vi "Module_UI_TopLevel.vi"(8 "error in (no error)":errorcluster, 10 "Wait on Module(s) (\"\": none)":string, 11 "ConfigFiles Folder Path":path) -> (0 "error out":errorcluster)   [LabVIEW 2019, in "Module_UI_TopLevel.lvclass"]
doc: "JSMA Module Template - Top Level UI 0.2.0.4\nRob Humfeld - Jet Engineering\nCopyright (c) 2019, Jet Engineering"
uses:
  Module_UI_TopLevel.lvclass
  Private/Module_UI_TopLevel_JETLogo STYP.ctl
  XControl_Menu Button/Menu Button.xctl
  Private/Module_UI_TopLevel_SPRight STYP.ctl
  Private/Module_UI_TopLevel_SPBottom STYP.ctl
  Private/Module_UI_TopLevel_SPCenter STYP.ctl
  C:/Program Files/National Instruments/LabVIEW 2019/user.lib/Jet Engineering/JSMA/Libraries/jModule Class/jModule.lvclass
  Private/Module_UI_TopLevel_jMsgTx STYP.ctl
  <userlib>/Jet Engineering/JSMA/Libraries/jMsg_CORE/jMsg_JSMA_ApplicationShutdown/jMsg_JSMA_ApplicationShutdown.lvclass
  C:/Program Files/National Instruments/LabVIEW 2019/user.lib/Jet Engineering/JSMA/Libraries/jMsg Class/jMsg.lvclass
  <userlib>/JET Engineering/JSMA Standard Messages/jMsg_Sys_UIPanelOpen/jMsg_Sys_UIPanel_Open.lvclass
  <userlib>/Jet Engineering/JSMA GUISubPanel CORE/jMsgs/jMsg_Sys_GUIPanelDock/jMsg_GUISubPanel_Dock.lvclass
  <userlib>/Jet Engineering/JSMA GUISubPanel CORE/jMsgs/jMsg_Sys_GUIPanelUndocked/jMsg_GUISubPanel_Undocked.lvclass
  Private/Module_UI_TopLevel_jMsgRx STYP.ctl
  <userlib>/Jet Engineering/JSMA Standard Messages/jMsg_Sys_VersionInfo/jMsg_Sys_VersionInfo.lvclass
  Private/Module_UI_TopLevel_Status STYP.ctl
  Module_UI_TopLevel.lvclass/Module_UI_TopLevel.ctl
  <userlib>/Jet Engineering/JSMA/Libraries/jModule Class/jModule.lvclass/jModule.ctl
  <userlib>/Jet Engineering/JSMA/Libraries/jMsg Class/jMsg.lvclass/jMsg.ctl
  <userlib>/JET Engineering/JSMA Standard Messages/jMsg_Sys_UIPanelOpen/jMsg_Sys_UIPanel_Open.lvclass/jMsg_Sys_UIPanel_Open.ctl
  <userlib>/Jet Engineering/JSMA/Libraries/jMsg_CORE/jMsg_JSMA_Exception/jMsg_JSMA_Exception.lvclass/jMsg_JSMA_Exception.ctl
  <userlib>/Jet Engineering/JSMA/Libraries/jMsg_CORE/jMsg_JSMA_SubscriptionChange/jMsg_JSMA_SubscriptionChange.lvclass/jMsg_JSMA_SubscriptionChange.ctl
  <userlib>/Jet Engineering/JSMA/Libraries/jMsg_CORE/jMsg_Addressed/jMsg_Addressed.lvclass/jMsg_Addressed.ctl
  <userlib>/Jet Engineering/JSMA/Libraries/jMsg_CORE/jMsg_JSMA_ApplicationShutdown/jMsg_JSMA_ApplicationShutdown.lvclass/jMsg_JSMA_ApplicationShutdown.ctl
  <userlib>/Jet Engineering/JSMA GUISubPanel CORE/jMsgs/jMsg_Sys_GUIPanelDock/jMsg_GUISubPanel_Dock.lvclass/jMsg_GUISubPanel_Dock.ctl
  <userlib>/Jet Engineering/JSMA Standard Messages/jMsg_Sys_VersionInfo/jMsg_Sys_VersionInfo.lvclass/jMsg_Sys_VersionInfo.ctl
  <userlib>/Jet Engineering/JET_QSM/Code/Private/JET_QSM - Add State [String API].vi
  <userlib>/Jet Engineering/JET_QSM/Code/Private/JET_QSM - Add State to Front [String API].vi
  <userlib>/Jet Engineering/JSMA/Libraries/jModule Class/jModule - Set Static Timer.vi
  <userlib>/Jet Engineering/JSMA/Libraries/jModule Class/jModule - Set Periodic Timer.vi
  <userlib>/Jet Engineering/JSMA/Libraries/jMsg Class/(create) jMsg.vi
  <userlib>/Jet Engineering/JSMA/Libraries/jMsg_CORE/jMsg_JSMA_Exception/(create) jMsg_JSMA_Exception.vi
  <userlib>/Jet Engineering/JSMA/Libraries/jModule Class/jModule - Stats_Exception Count Increment.vi
  <userlib>/Jet Engineering/JSMA/Libraries/jModule Class/jModule - SimpleTx.vi
  <userlib>/Jet Engineering/JSMA/Libraries/jModule Class/jModule - Exception Enqueue.vi
  <userlib>/Jet Engineering/JSMA/Libraries/jMsg Class/Read No Listener Action.vi
  <userlib>/Jet Engineering/JSMA/Libraries/jModule Class/jModule - ExceptionBatchTx.vi
  <userlib>/Jet Engineering/JSMA/Libraries/jModule Class/jModule - Send to List.vi
  <userlib>/Jet Engineering/JSMA/Libraries/jModule Class/jModule - AddressedTx.vi
  <userlib>/Jet Engineering/JSMA/Libraries/jModule Class/jModule - Stats_Tx Count Increment.vi
  <userlib>/Jet Engineering/JSMA/Libraries/jMsg Class/Read Type.vi
  <userlib>/Jet Engineering/JSMA/Libraries/jMsg Class/Write SendID.vi
  <userlib>/Jet Engineering/JSMA/Libraries/jMsg Class/Read Name.vi
  <userlib>/Jet Engineering/JSMA/Libraries/jMasterTable_Subscription/jMasterTable_Subscription - Get Queue Type.vi
  <userlib>/Jet Engineering/JSMA/Libraries/jMsg Class/jMsg - Set Source.vi
  <userlib>/Jet Engineering/JSMA/Libraries/jMasterShutdownFlag/jFlag_MasterShutdown - Set.vi
  <userlib>/Jet Engineering/JSMA/Libraries/jModule Class/Read jMsgRx.vi
  <userlib>/Jet Engineering/JSMA/Libraries/Shared/JSMA_GetClassName.vi
  <userlib>/Jet Engineering/JSMA/Libraries/jMsg Class/Read Sent Time.vi
  <userlib>/Jet Engineering/JSMA/Libraries/jMsg Class/Read Source.vi
  <userlib>/Jet Engineering/JSMA/Libraries/jMasterTable_Subscription/jMasterTable_Subscription - Remove Module.vi
  <userlib>/Jet Engineering/JSMA/Libraries/jMsg Class/Write Source.vi
  <userlib>/Jet Engineering/JSMA/Libraries/jMsg_CORE/jMsg_JSMA_SubscriptionChange/(create) jMsg_JSMA_SubscriptionChange.vi
  <userlib>/Jet Engineering/JSMA/Libraries/jMasterTable_Subscription/jMasterTable_Subscription - Get Sub List.vi
  <userlib>/Jet Engineering/JSMA/Libraries/jMsg_CORE/jMsg_Addressed/Read Qualified Name.vi
  <userlib>/Jet Engineering/JSMA/Libraries/jMsg_CORE/jMsg_Addressed/Read RecvID.vi
  <userlib>/Jet Engineering/JSMA/Libraries/jMasterTable_Subscription/jMasterTable_Subscription - Get-Create Queue.vi
  <userlib>/Jet Engineering/JSMA/Libraries/jMasterTable_Message/jMasterTable_Message - Add jMsg.vi
  <userlib>/Jet Engineering/JSMA/Libraries/jMasterTable_Message/jMasterTable_Message - Get-Create Queue.vi
  <userlib>/Jet Engineering/JSMA/Libraries/jMsg_CORE/jMsg_JSMA_Exception/jMsg_JSMA_Exception.lvclass
  <userlib>/Jet Engineering/JSMA/Libraries/jMsg_CORE/jMsg_JSMA_SubscriptionChange/jMsg_JSMA_SubscriptionChange.lvclass
  <userlib>/Jet Engineering/JSMA/Libraries/jMsg_CORE/jMsg_Addressed/jMsg_Addressed.lvclass
  <vilib>/Utility/error.llb/Trim Whitespace.vi
  <vilib>/Utility/LVClass/Get LV Class Path.vi
  <userlib>/Jet Engineering/JSMA/Libraries/jMasterShutdownFlag/jFlag_MasterShutdown_FGV.vi
  <vilib>/Utility/error.llb/Error Cluster From Error Code.vi
  <userlib>/Jet Engineering/JSMA/Libraries/jModule Class/Read RxQueue.vi
  <userlib>/Jet Engineering/JSMA/Libraries/jSubscription Class/jSubscription.lvclass
  <userlib>/Jet Labs/JET Panel/JETPanel.lvclass
  <userlib>/Jet Engineering/JSMA/Libraries/jModule Class/jModule.lvclass
  <userlib>/Jet Engineering/JSMA/Libraries/jMasterShutdownFlag/jFlag_MasterShutdown.lvclass
  <userlib>/Jet Engineering/JSMA/Libraries/jMsg Class/jMsg.lvclass
panel:
  out "Center":T1=enum."Module_SP_CenterBlank#5"
  out "Bottom":T2=enum."Module_SP_BottomBlank#6"
  out "Right":T3=enum."Module_SP_RightBlank#7"
  out "Menu Level":string
  out "Menu Button":string
  out "String":string
  out "TCPStats":string
  out "FPGA":string caption="FPGA IO:"
  out "Host":string caption="Host PC:"
  in  "Menu":T4(xcontrol)
  in  "JET":T5
  out "currentDateTime":dbl format="%<%m/%d/%y %H:%M:%S>T"
  in  "exit?":bool
  out "winSizer 2":string="W"
  out "winSizer 1":string="W"
  out "Recent states before Error (with tick counts) 2":string="0.167 sec ago: VI Initialize\n0.167 sec ago: Window Open\n0.110 sec ago: Control Update\n0.110 sec ago: Indicator Update\n0.000 sec ago: Error Handler\r\n"
  out "Header":bool
  out "JETLogo":bool
  # "LOGO"
  # "LOGO"
  # "Project Name"
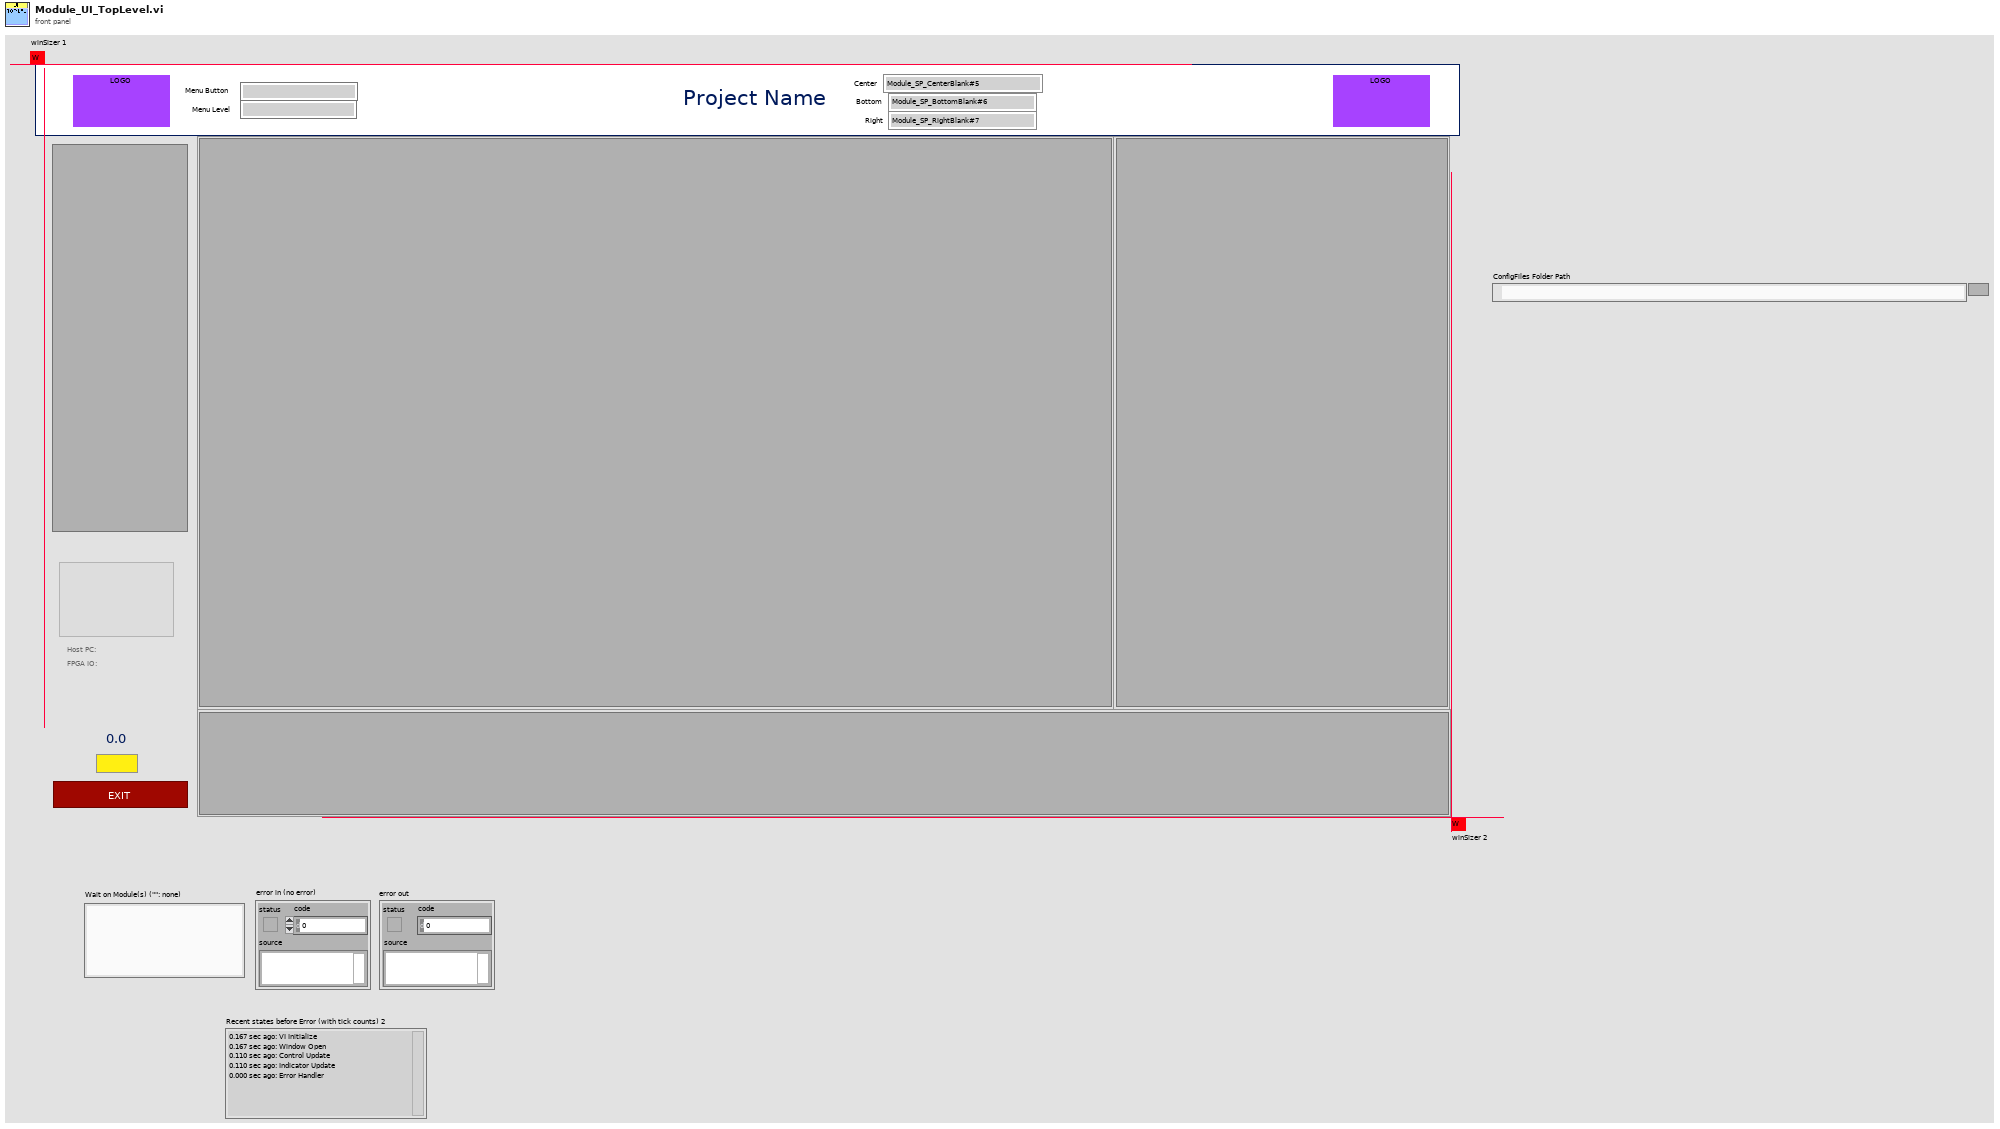
[diagram p1: front panel]
types:
  T1 = typedef "Module_UI_TopLevel.lvclass/Module_UI_TopLevel_SPCenter STYP.ctl" = enum16{"Module_SP_GameDisplay#0", "Module_SP_CenterBlank#5", "Module_SP_SALSignalConfig#4", "Module_SP_TestConfiguration#10", "Module_SP_TestExecution#9"}
  T2 = typedef "Module_UI_TopLevel.lvclass/Module_UI_TopLevel_SPBottom STYP.ctl" = enum16{"Module_SP_GameStats#2", "Module_SP_BottomBlank#6", "Module_SP_StatusRibbon#8"}
  T3 = typedef "Module_UI_TopLevel.lvclass/Module_UI_TopLevel_SPRight STYP.ctl" = enum16{"Module_SP_GameLeaderboard#1", "Module_SP_RightBlank#7", "Module_SP_SystemEventLog"}
  T4 = cluster{"Button Pressed":string, "Level":string, "Menu Config":variant}
  T5 = typedef "Module_UI_TopLevel.lvclass/Module_UI_TopLevel_JETLogo STYP.ctl" = bool
  T6 = typedef "Module_UI_TopLevel.lvclass/Module_UI_TopLevel_jMsgRx STYP.ctl" = cluster{"Msg_Sys_VersionInfo":refnum<class "jMsg_Sys_VersionInfo.lvclass">, "jMsg_GUISubPanel_Dock":refnum<class "jMsg_GUISubPanel_Dock.lvclass">}
  T7 = typedef "Module_UI_TopLevel.lvclass/Module_UI_TopLevel_jMsgTx STYP.ctl" = cluster{"jMsg_JSMA_ApplicationShutdown":refnum<class "jMsg_JSMA_ApplicationShutdown.lvclass">, "jMsg_Sys_UIPanel_Open":refnum<class "jMsg_Sys_UIPanel_Open.lvclass">, "jMsg_GUISubPanel_Dock":refnum<class "jMsg_GUISubPanel_Dock.lvclass">, "jMsg_GUISubPanel_Undocked":refnum<class "jMsg_GUISubPanel_Undocked.lvclass">}
  T8 = typedef "Module_UI_TopLevel.lvclass/Module_UI_TopLevel_Status STYP.ctl" = cluster{"VI":cluster{"error":errorcluster, "isExiting?":bool}, "UI":cluster{"SP_center":cluster{"refnum":refnum<vi>, "ActivePanel":T1}, "SP_bottom":cluster{"refnum":refnum<vi>, "ActivePanel":T2}, "SP_right":cluster{"refnum":refnum<vi>, "ActivePanel":T3}}, "TCPConnected?":bool}
  T9 = typedef "JET_QSM_Refnum STYP.ctl" = cluster{"state":cluster{"queue":refnum<queue>, "idle":string, "error":string, "STOP":string}, "debug":cluster{"enabled?":bool, "queue":refnum<queue>}, "Invalid.option":T10, "QSM.Name":string}
  T10 = typedef "JET_QSM_InvalidOption STYP.ctl" = enum16{"Ignore", "Dialog", "Error"}
  T11 = typedef "eventvkey.ctl" = enum16{"ASCII", "Enter", "Return", "Shift", "Ctrl", "Alt", "Cmd", "Opt", "Caps", "NumLock", "Clear", "Break", "Up", "Down", "Left", "Right", "Insert", "Delete", "Home", "End", "PageUp", "PageDown", "Escape", "Help", "Pause", "ScrollLock", "F1", "F2", "F3", "F4", "F5", "F6", "F7", "F8", "F9", "F10", "F11", "F12", "F13", "F14", "F15", "F16", "F17", "F18", "F19", "F20", "F21", "F22", "F23", "F24", "Play", "VolumeUp", "VolumeDown", "Mute", "Two Byte Char"}
  T12 = cluster{"Shift":bool, "Ctrl":bool, "Alt":bool, "Cmd":bool, "Opt":bool}
  T13 = typedef "JET_QSM_Element STYP.ctl" = cluster{"state":string, "data":variant, "comment":string}
  T14 = typedef "JSMAjMsg_Standard.lvlib/jMsg_Sys_VersionInfo.lvclass/VersionInfo STYP.ctl" = cluster{"ID":string, "Version":string, "Date":string}
  T15 = typedef "jSWCfg_SoftwareInfo STYP.ctl" = cluster{"target ID":string, "version":string, "releaseDate":string}
  T16 = enum8{"Enabled", "Disabled", "Disabled and Grayed Out"}
  T17 = typedef "jSWCfg_PROPERTIES STYP.ctl" = cluster{"SoftwareID":string, "SoftwareInfo.array":T15[]}
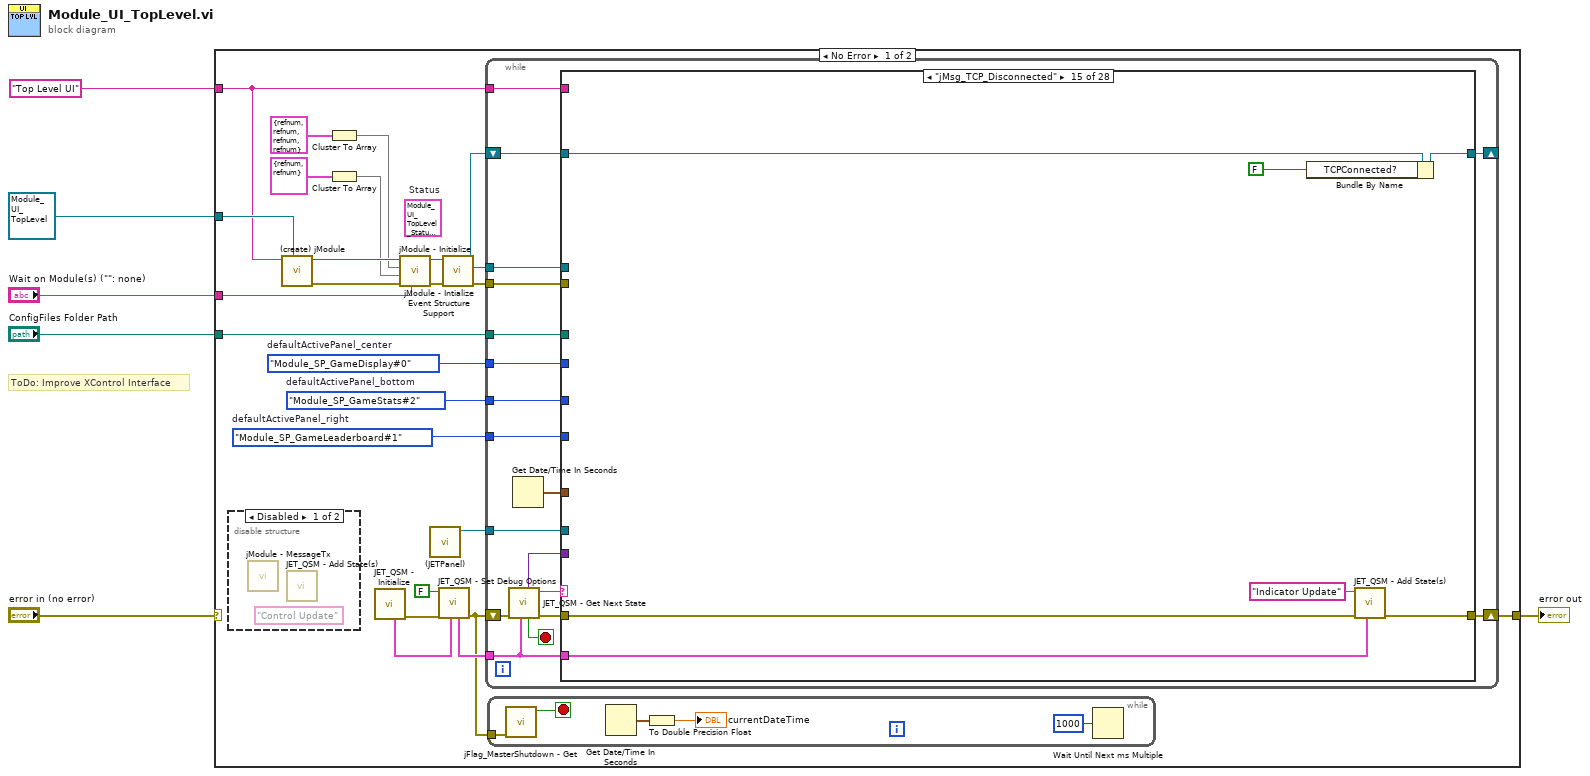
[diagram p0: block diagram]
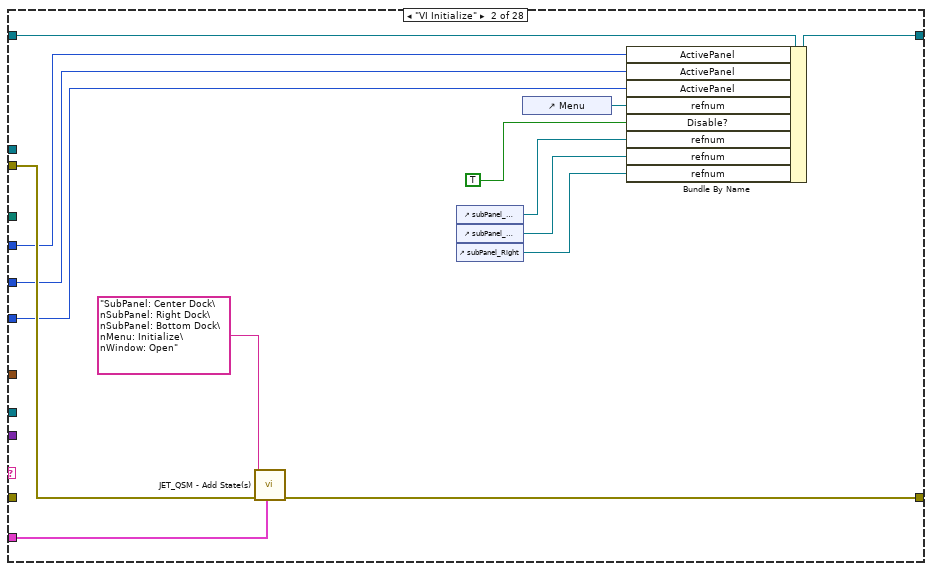
[diagram p4: hidden frame]
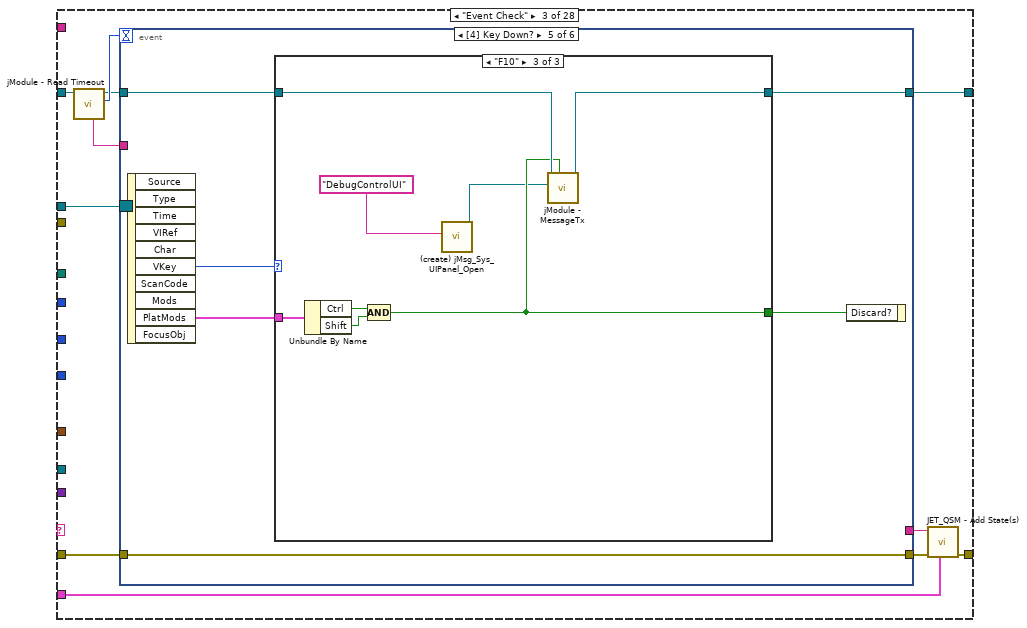
[diagram p5: hidden frame]
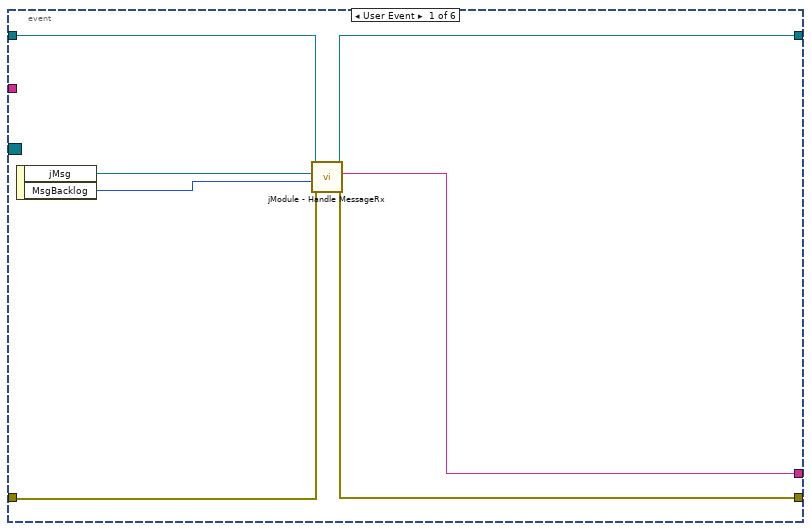
[diagram p6: hidden frame]
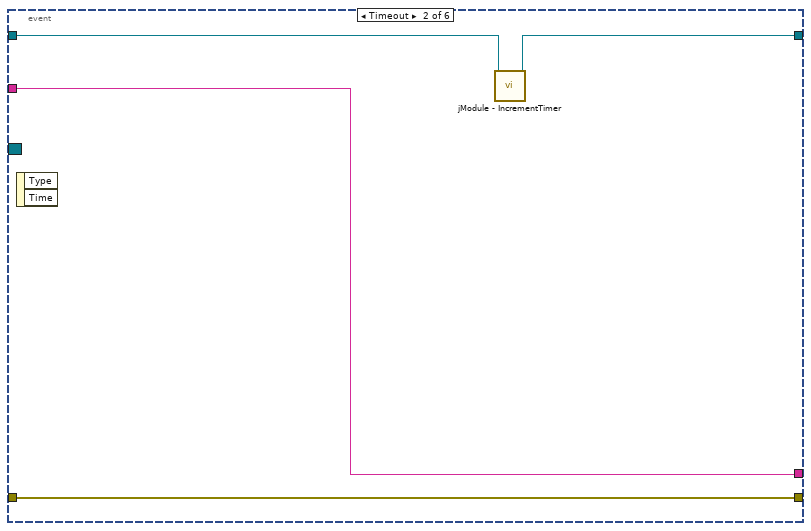
[diagram p7: hidden frame]
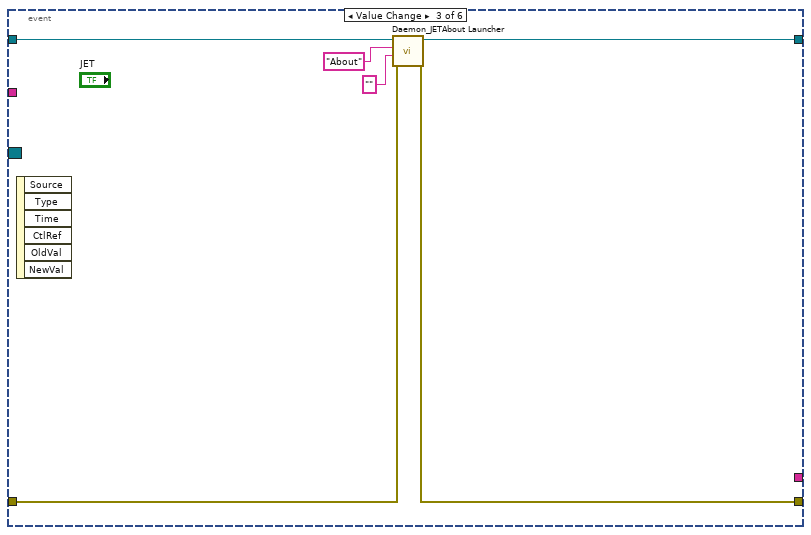
[diagram p8: hidden frame]
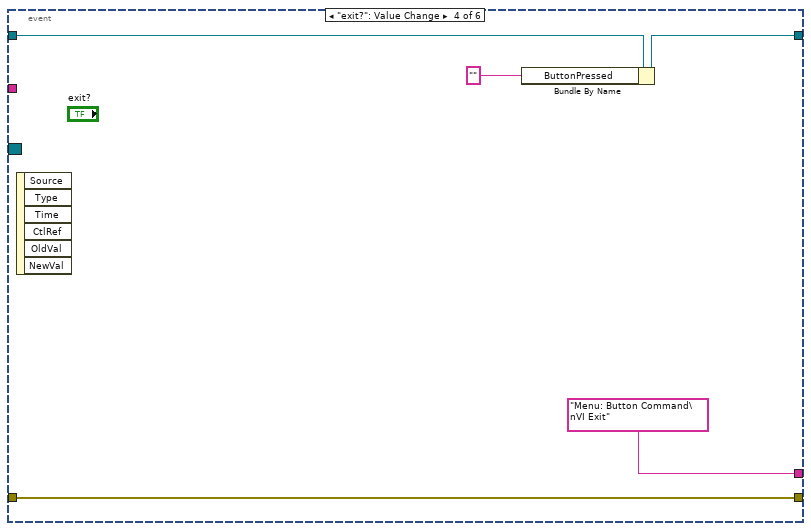
[diagram p9: hidden frame]
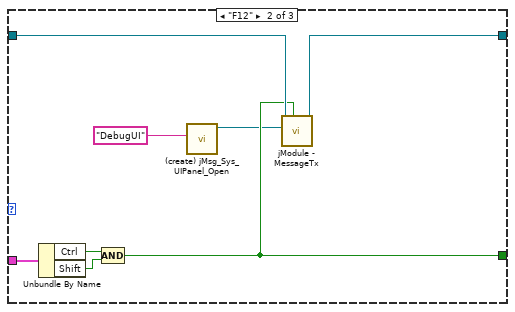
[diagram p11: hidden frame]
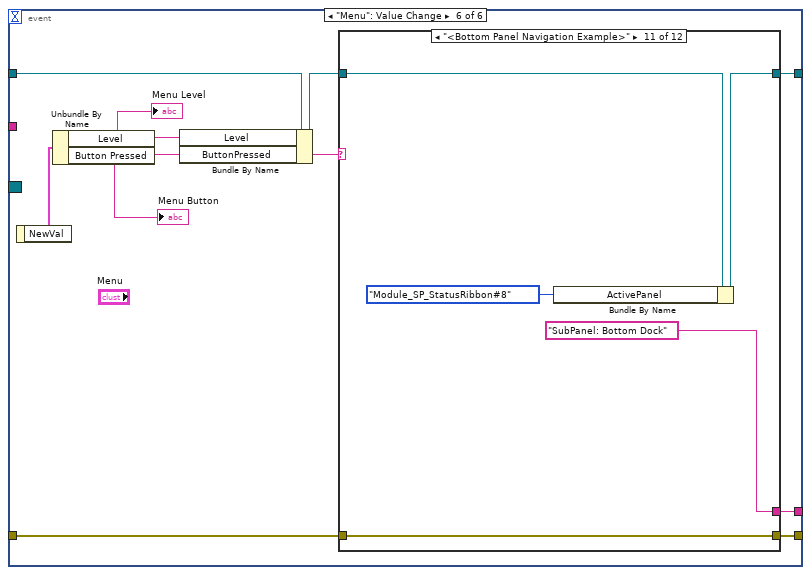
[diagram p12: hidden frame]
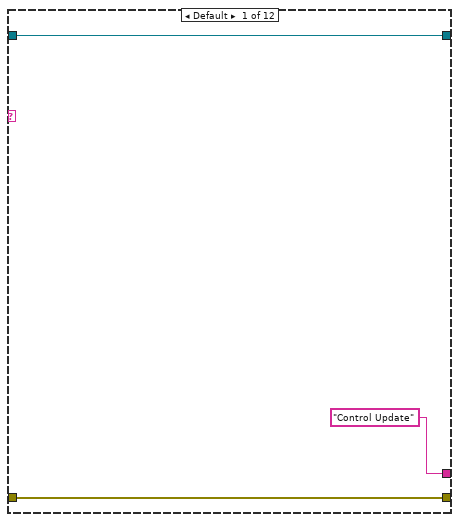
[diagram p13: hidden frame]
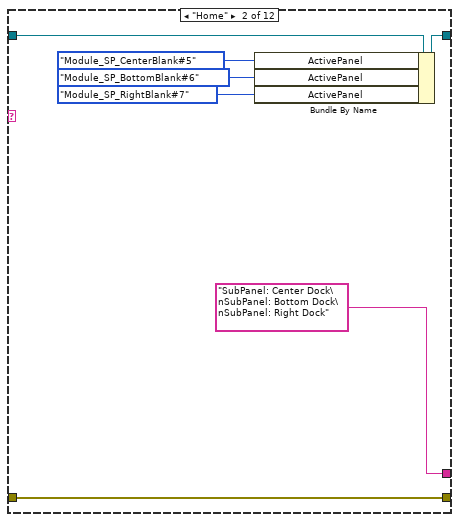
[diagram p14: hidden frame]
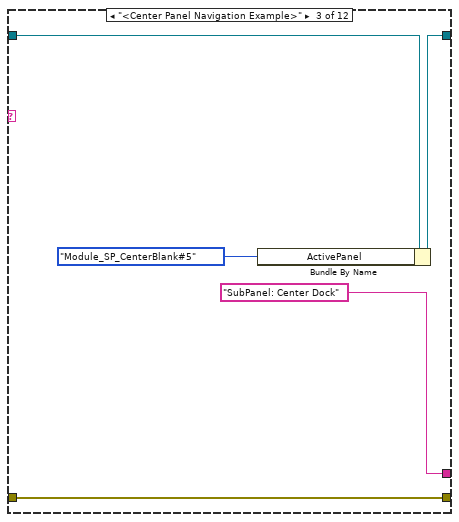
[diagram p15: hidden frame]
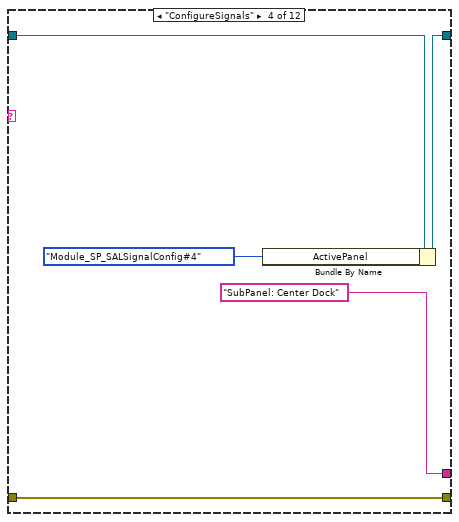
[diagram p16: hidden frame]
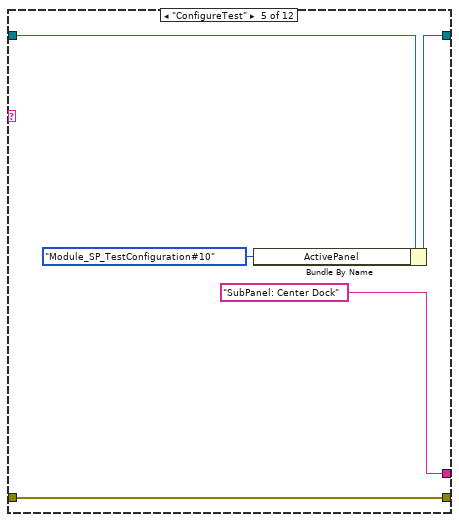
[diagram p17: hidden frame]
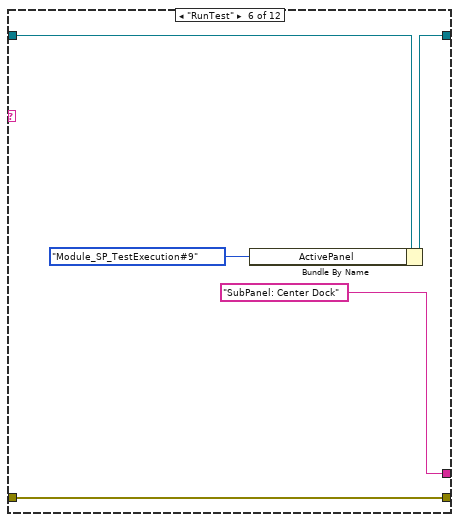
[diagram p18: hidden frame]
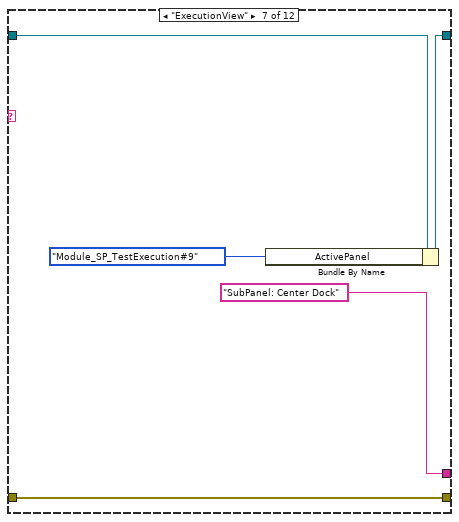
[diagram p19: hidden frame]
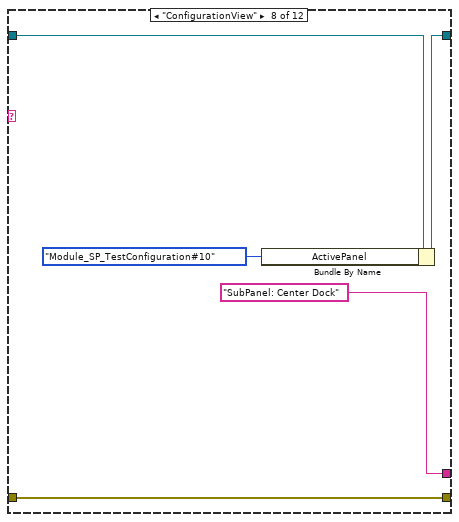
[diagram p20: hidden frame]
diagram:
  # "ToDo: Improve XControl Interface"
  n1 = case shown="No Error" "error in (no error)" {
    selector: "error in (no error)" -> [_ w426]
    tunnel: [w31 w426] -> w6
    tunnel: "Wait on Module(s) (\"\": none)" -> [w17 _]
    tunnel: "Top Level UI" ("jModule Name (\"\": use calling VI's name)") -> [w10 _]
    tunnel: refnum<class "Module_UI_TopLevel.lvclass"> refnum ("Module_UI_TopLevel.lvclass") -> [w13 _]
    tunnel: "ConfigFiles Folder Path" -> [w11 _]
    frame No Error {
      w8 = Module_UI_TopLevel_SPBottom_STYP."Module_SP_GameStats#2"  # defaultActivePanel_bottom
      w9 = Module_UI_TopLevel_SPCenter_STYP."Module_SP_GameDisplay#0"  # defaultActivePanel_center
      w7 = Module_UI_TopLevel_SPRight_STYP."Module_SP_GameLeaderboard#1"  # defaultActivePanel_right
      (unwired) T8 {"VI"={"error"={"status"=FALSE, "code"=0, "source"=""}, "isExiting?"=FALSE}, "UI"={"SP_center"={"refnum"=refnum, "ActivePanel"=enum."Module_SP_CenterBlank#5"}, "SP_bottom"={"refnum"=refnum, "ActivePanel"=enum."Module_SP_BottomBlank#6"}, "SP_right"={"refnum"=refnum, "ActivePanel"=enum."Module_SP_RightBlank#7"}}, "TCPConnected?"=FALSE}  # Status
      n2 = disable-structure shown="Disabled" {
        frame Disabled {
          (unwired) "Control Update"
          n3 = call <userlib>:"jModule - MessageTx.vi"() -> ()  [unwired: 8 in, 4 out]
          n4 = call-poly <userlib>:"JET_QSM - Add State(s).vi"() -> ()  [unwired: 11 in, 1 out]
        }
        frame Enabled {
        }
      }
      n5 = call <userlib>:"(create) jModule.vi"("jModule Child class"=w13, "jModule Name (\"\": use calling VI's name)"=w10) -> ("error out"=w23:errorcluster, "jModule"=w25:refnum<class "Module_UI_TopLevel.lvclass">)  [unwired: 6 in, 2 out]
      n6 = Cluster To Array(cluster=T7 {"jMsg_JSMA_ApplicationShutdown"=refnum, "jMsg_Sys_UIPanel_Open"=refnum, "jMsg_GUISubPanel_Dock"=refnum, "jMsg_GUISubPanel_Undocked"=refnum} ("TxMsg")) -> (array=w24:refnum<class "jMsg.lvclass">[])
      n7 = Cluster To Array(cluster=T6 {"Msg_Sys_VersionInfo"=refnum, "jMsg_GUISubPanel_Dock"=refnum} ("RxMsg")) -> (array=w19:refnum<class "jMsg.lvclass">[])
      n8 = call <userlib>:"JET_QSM - Initialize.vi"() -> ("error out"=w27:errorcluster, "Jet_QSM refnum"=w29:T9)  [unwired: 10 in]
      n9 = call-dynamic "jModule - Initialize.vi"("Wait on Module(s) (\"\": none)"=w17, "error in (no error)"=w23, "jMsgRxList"=w19, "jMsgTxList"=w24, "jModule"=w25) -> ("error out"=w22:errorcluster, "jModule"=w21:refnum<class "Module_UI_TopLevel.lvclass">)  [unwired: 5 in]
      n10 = call <userlib>:"(JETPanel).vi"() -> ("JETPanel"=w26:refnum<class "JETPanel.lvclass">)  [unwired: 8 in, 3 out]
      n11 = call <userlib>:"JET_QSM - Set Debug Options.vi"("Jet_QSM refnum"=w29, "error in (no error)"=w27, "debug.enabled? (F)"=FALSE) -> ("error out"=w16:errorcluster, "Jet_QSM ref"=w28:T9)  [unwired: 7 in]
      n12 = call <userlib>:"jModule - Intialize Event Structure Support.vi"("error in (no error)"=w22, "jModule"=w21) -> ("error out"=w18:errorcluster, "Event Registration Refnum"=w20:refnum<event-registration>, "jModule"=w12:refnum<class "Module_UI_TopLevel.lvclass">)  [unwired: 6 in, 1 out]
      n13 = while {
        tunnel: w28 -> [w50]
        shift-right: [w37] -> _
        shift-left: w12 -> [w49]
        shift-right: [w48] -> w31
        shift-left: w16 -> [w54]
        tunnel: w26 -> [w47]
        tunnel: w18 -> [w46]
        tunnel: w20 -> [w45]
        tunnel: w10 -> [w44]
        tunnel: w11 -> [w41]
        tunnel: w9 -> [w40]
        tunnel: w8 -> [w39]
        tunnel: w7 -> [w38]
        stop <- w51 stop-if-true
        n14 = call <userlib>:"JET_QSM - Get Next State.vi"("Jet_QSM refnum"=w50, "error in (no error)"=w54) -> ("error out"=w53:errorcluster, "state"=w52:string, "Stop Loop?"=w51:bool, "state data"=w43:variant)  [unwired: 5 in, 1 out]
        n15 = Get Date/Time In Seconds() -> (seconds since 1Jan1904=w42:timestamp)
        n16 = case shown="\"jMsg_TCP_Disconnected\"" w52 {
          selector: w52 -> [_ _ _ _ _ _ w246 _ _ _ _ _ _ _ _ _ _ _ _ _ _ _ _ _ _ _ _ _]
          tunnel: w53 -> [w55 _ w81 w198 w229 _ w247 w256 w258 w260 w275 w297 w310 w317 w324 w327 w334 w341 w347 w360 w367 w374 w375 w379 w393 w397 w416 w424]
          tunnel: w50 -> [_ w70 w80 w202 w228 _ w244 _ _ w264 _ w304 w312 w314 w321 _ _ _ _ _ _ _ _ _ w394 _ w417 _]
          tunnel: w49 -> [w56 w61 w72 w197 w223 w239 w243 w257 w259 w261 w266 w298 w306 w319 w326 w328 w332 w340 w350 w354 w361 w368 w376 w380 w390 w396 w418 w425]
          tunnel: [w56 w67 w76 w196 w226 w239 w242 w257 w259 w261 w269 w295 w305 w318 w325 w328 w331 w340 w353 w355 w362 w373 w376 w380 w390 w396 w418 w425] -> w37
          tunnel: [w55 w69 w78 w203 _ w241 w245 w256 w258 w263 w275 w303 w309 w316 w323 w327 w333 w341 w344 w360 w367 w374 w375 w379 w392 w397 w415 w424] -> w48
          tunnel: w47 -> [_ _ _ _ _ w240 _ _ _ _ _ _ _ _ _ _ _ _ _ _ _ _ _ _ _ _ w413 w423]
          tunnel: w46 -> [_ w68 _ _ _ _ _ _ _ _ _ _ _ _ _ _ _ _ _ _ _ _ _ _ _ _ _ _]
          tunnel: w45 -> [_ _ w75 _ _ _ _ _ _ _ _ _ _ _ _ _ _ _ _ _ _ _ _ _ _ _ _ _]
          tunnel: w44 -> [_ _ _ _ _ _ _ _ _ _ _ w301 _ _ _ _ _ _ _ _ _ _ _ _ _ _ w409 _]
          tunnel: w43 -> [_ _ _ _ _ _ _ _ _ _ _ _ _ _ _ _ _ _ _ _ _ _ _ _ _ _ _ _]
          tunnel: w42 -> [_ _ _ _ _ _ _ _ _ _ _ _ _ _ _ _ _ _ _ _ _ _ _ _ _ _ _ _]
          tunnel: w41 -> [_ _ _ _ _ _ _ _ _ _ _ _ _ _ _ _ _ _ w351 _ _ _ _ _ _ _ _ _]
          tunnel: w40 -> [_ w59 _ _ _ _ _ _ _ _ _ _ _ _ _ _ _ _ _ _ _ _ _ _ _ _ _ _]
          tunnel: w39 -> [_ w58 _ _ _ _ _ _ _ _ _ _ _ _ _ _ _ _ _ _ _ _ _ _ _ _ _ _]
          tunnel: w38 -> [_ w57 _ _ _ _ _ _ _ _ _ _ _ _ _ _ _ _ _ _ _ _ _ _ _ _ _ _]
          frame "------ Standard States ------" {
            # "Standard States are required states for a JET_QSM State Machine\n\nTheir names may be changed; use the Initialize function to specify the new names"
            # "This is a section header; the state is never expected to execute"
          }
          frame "VI Initialize" {
            n17 = call-poly <userlib>:"JET_QSM - Add State(s).vi"("Jet_QSM refnum"=w70, "error in (no error)"=w68, "state(s)"="SubPanel: Center Dock\nSubPanel: Right Dock\nSubPanel: Bottom Dock\nMenu: Initialize\nWindow: Open") -> ("error out"=w69:errorcluster)  [unwired: 8 in]
            n18 = control-ref of="subPanel_Center"() -> (w64:refnum<vi>)
            n19 = control-ref of="subPanel_Bottom"() -> (w63:refnum<vi>)
            n20 = control-ref of="subPanel_Right"() -> (w62:refnum<vi>)
            n21 = control-ref of="Menu"() -> (w60:refnum<vi>)
            n22 = Bundle By Name(cluster=w61, "ActivePanel"=w59, "ActivePanel"=w58, "ActivePanel"=w57, "refnum"=w60, "Disable?"=TRUE ("Settings.MenuDisable?"), "refnum"=w64, "refnum"=w63, "refnum"=w62) -> (w67:refnum<class "Module_UI_TopLevel.lvclass">)
          }
          frame "Event Check" {
            n23 = call <userlib>:"jModule - Read Timeout.vi"("jModule"=w72) -> ("Timeout, ms"=w74:i32, "jModule"=w71:refnum<class "Module_UI_TopLevel.lvclass">, "Timeout.State"=w73:string)  [unwired: 8 in]
            n24 = event shown="[4] Key Down?" {
              selector: w75 -> [_ _ _ _ _ _]
              dyn-events: _ -> [_ _ _ _ _ _]
              timeout: w74 -> [_ _ _ _ _ _]
              tunnel: w81 -> [w86 w91 w98 w103 w109 w133]
              tunnel: [w87 w92 _ "Menu: Button Command\nVI Exit" ("Timeout.State") _ w131] -> w79
              tunnel: [w85 w91 w97 w103 w109 w132] -> w77
              tunnel: w71 -> [w83 w90 w94 w100 w105 w130]
              tunnel: [w82 w89 w93 w102 w104 w128] -> w76
              tunnel: w73 -> [_ w92 _ _ _ _]
              event User Event {
                n25 = event-data() -> ("jMsg"=w88:refnum<class "jMsg.lvclass">, "MsgBacklog"=w84:i32)  [unwired: 1 in]
                n26 = call-dynamic "jModule - Handle MessageRx.vi"("error in (no error)"=w86, "Message Backlog"=w84, "jMsg"=w88, "jModule"=w83) -> ("error out"=w85:errorcluster, "QSMState"=w87:string, "jModule"=w82:refnum<class "Module_UI_TopLevel.lvclass">)  [unwired: 4 in, 1 out]
              }
              event Timeout {
                n27 = event-data() -> ()  [unwired: 1 in, 2 out]
                n28 = call <userlib>:"jModule - IncrementTimer.vi"("jModule"=w90) -> ("jModule"=w89:refnum<class "Module_UI_TopLevel.lvclass">)  [unwired: 10 in]
              }
              event Value Change {
                n29 = event-data() -> ()  [unwired: 1 in, 6 out]
                n30 = call "Daemon_JETAbout Launcher.vi"("error in"=w98, "Dialog Text"="", "Dialog Name"="About", "jModule"=w94) -> ("error out"=w97:errorcluster, "jModule"=w93:refnum<class "Module_UI_TopLevel.lvclass">)  [unwired: 5 in, 1 out]
              }
              event "exit?": Value Change {
                n31 = event-data() -> ()  [unwired: 1 in, 6 out]
                n32 = Bundle By Name(cluster=w100, "ButtonPressed"="" ("MenuButton.New")) -> (w102:refnum<class "Module_UI_TopLevel.lvclass">)
              }
              event Key Down? {
                n33 = event-data() -> ("VKey"=w106:T11, "PlatMods"=w108:T12)  [unwired: 1 in, 8 out]
                n34 = case shown="\"F10\"" w106 {
                  tunnel: w108 -> [_ w118 w126]
                  tunnel: [_ w113 w121] -> w107
                  tunnel: w105 -> [w110 w114 w122]
                  tunnel: [w110 w115 w123] -> w104
                  frame Default {
                  }
                  frame "F12" {
                    n35 = Unbundle By Name(w118) -> ("Ctrl"=w117:bool, "Shift"=w116:bool)
                    n36 = Compound Arithmetic op=AND(w117, w116) -> (w113:bool)
                    n37 = call <userlib>:"(create) jMsg_Sys_UIPanel_Open.vi"("UI Name"="DebugUI" ("GUI")) -> ("jMsg_Sys_UIPanel_Open"=w112:refnum<class "jMsg_Sys_UIPanel_Open.lvclass">)  [unwired: 10 in]
                    n38 = call <userlib>:"jModule - MessageTx.vi"("Act? (T)"=w113, "jMsg"=w112, "jModule"=w114) -> ("jModule"=w115:refnum<class "Module_UI_TopLevel.lvclass">)  [unwired: 5 in, 3 out]
                  }
                  frame "F10" {
                    n39 = Unbundle By Name(w126) -> ("Ctrl"=w125:bool, "Shift"=w124:bool)
                    n40 = Compound Arithmetic op=AND(w125, w124) -> (w121:bool)
                    n41 = call <userlib>:"(create) jMsg_Sys_UIPanel_Open.vi"("UI Name"="DebugControlUI" ("GUI")) -> ("jMsg_Sys_UIPanel_Open"=w119:refnum<class "jMsg_Sys_UIPanel_Open.lvclass">)  [unwired: 10 in]
                    n42 = call <userlib>:"jModule - MessageTx.vi"("Act? (T)"=w121, "jMsg"=w119, "jModule"=w122) -> ("jModule"=w123:refnum<class "Module_UI_TopLevel.lvclass">)  [unwired: 5 in, 3 out]
                  }
                }
                n43 = event-data("Discard?"=w107) -> ()  [unwired: 1 in, 1 out]
              }
              event "Menu": Value Change {
                n44 = event-data() -> ("NewVal"=w127:T4)  [unwired: 1 in]
                n45 = Unbundle By Name(w127) -> ("Level"=w135:string, "Button Pressed"=w134:string)
                "Menu Button" <- w134
                "Menu Level" <- w135
                n46 = Bundle By Name(cluster=w130, "Level"=w135, "ButtonPressed"=w134) -> (w129:refnum<class "Module_UI_TopLevel.lvclass">)
                n47 = case shown="\"<Bottom Panel Navigation Example>\"" w134 {
                  tunnel: w133 -> [w138 w145 w150 w155 w160 w165 w170 w175 w180 w185 w190 w195]
                  tunnel: [w138 w145 w150 w155 w160 w165 w170 w175 w180 w185 w190 w195] -> w132
                  tunnel: [w136 w142 w147 w152 w157 w162 w167 w172 w177 w182 w187 w192] -> w128
                  tunnel: ["Control Update" ("Timeout.State") "SubPanel: Center Dock\nSubPanel: Bottom Dock\nSubPanel: Right Dock" ("state(s)") "SubPanel: Center Dock" ("state(s)") "SubPanel: Center Dock" ("state(s)") "SubPanel: Center Dock" ("state(s)") "SubPanel: Center Dock" ("state(s)") "SubPanel: Center Dock" ("state(s)") "SubPanel: Center Dock" ("state(s)") "SubPanel: Right Dock" ("state(s)") "SubPanel: Right Dock" ("state(s)") "SubPanel: Bottom Dock" ("state(s)") "SubPanel: Bottom Dock" ("state(s)")] -> w131
                  tunnel: w129 -> [w136 w143 w148 w153 w158 w163 w168 w173 w178 w183 w188 w193]
                  frame Default {
                  }
                  frame "Home" {
                    n48 = Bundle By Name(cluster=w143, "ActivePanel"=Module_UI_TopLevel_SPCenter_STYP."Module_SP_CenterBlank#5" ("my.UI.SP_center.ActivePanel"), "ActivePanel"=Module_UI_TopLevel_SPBottom_STYP."Module_SP_BottomBlank#6" ("my.UI.SP_bottom.ActivePanel"), "ActivePanel"=Module_UI_TopLevel_SPRight_STYP."Module_SP_RightBlank#7" ("my.UI.SP_right.ActivePanel")) -> (w142:refnum<class "Module_UI_TopLevel.lvclass">)
                  }
                  frame "<Center Panel Navigation Example>" {
                    n49 = Bundle By Name(cluster=w148, "ActivePanel"=Module_UI_TopLevel_SPCenter_STYP."Module_SP_CenterBlank#5" ("my.UI.SP_center.ActivePanel")) -> (w147:refnum<class "Module_UI_TopLevel.lvclass">)
                  }
                  frame "ConfigureSignals" {
                    n50 = Bundle By Name(cluster=w153, "ActivePanel"=Module_UI_TopLevel_SPCenter_STYP."Module_SP_SALSignalConfig#4" ("my.UI.SP_center.ActivePanel")) -> (w152:refnum<class "Module_UI_TopLevel.lvclass">)
                  }
                  frame "ConfigureTest" {
                    n51 = Bundle By Name(cluster=w158, "ActivePanel"=Module_UI_TopLevel_SPCenter_STYP."Module_SP_TestConfiguration#10" ("my.UI.SP_center.ActivePanel")) -> (w157:refnum<class "Module_UI_TopLevel.lvclass">)
                  }
                  frame "RunTest" {
                    n52 = Bundle By Name(cluster=w163, "ActivePanel"=Module_UI_TopLevel_SPCenter_STYP."Module_SP_TestExecution#9" ("my.UI.SP_center.ActivePanel")) -> (w162:refnum<class "Module_UI_TopLevel.lvclass">)
                  }
                  frame "ExecutionView" {
                    n53 = Bundle By Name(cluster=w168, "ActivePanel"=Module_UI_TopLevel_SPCenter_STYP."Module_SP_TestExecution#9" ("my.UI.SP_center.ActivePanel")) -> (w167:refnum<class "Module_UI_TopLevel.lvclass">)
                  }
                  frame "ConfigurationView" {
                    n54 = Bundle By Name(cluster=w173, "ActivePanel"=Module_UI_TopLevel_SPCenter_STYP."Module_SP_TestConfiguration#10" ("my.UI.SP_center.ActivePanel")) -> (w172:refnum<class "Module_UI_TopLevel.lvclass">)
                  }
                  frame "<Right Panel Navigation Example>" {
                    n55 = Bundle By Name(cluster=w178, "ActivePanel"=Module_UI_TopLevel_SPRight_STYP."Module_SP_RightBlank#7" ("my.UI.SP_right.ActivePanel")) -> (w177:refnum<class "Module_UI_TopLevel.lvclass">)
                  }
                  frame "Save" {
                    n56 = Bundle By Name(cluster=w183, "ActivePanel"=Module_UI_TopLevel_SPRight_STYP."Module_SP_SystemEventLog" ("my.UI.SP_right.ActivePanel")) -> (w182:refnum<class "Module_UI_TopLevel.lvclass">)
                  }
                  frame "<Bottom Panel Navigation Example>" {
                    n57 = Bundle By Name(cluster=w188, "ActivePanel"=Module_UI_TopLevel_SPBottom_STYP."Module_SP_StatusRibbon#8" ("my.UI.SP_bottom.ActivePanel")) -> (w187:refnum<class "Module_UI_TopLevel.lvclass">)
                  }
                  frame "TestAbort" {
                    n58 = Bundle By Name(cluster=w193, "ActivePanel"=Module_UI_TopLevel_SPBottom_STYP."Module_SP_StatusRibbon#8" ("my.UI.SP_bottom.ActivePanel")) -> (w192:refnum<class "Module_UI_TopLevel.lvclass">)
                  }
                }
              }
            }
            n59 = call-poly <userlib>:"JET_QSM - Add State(s).vi"("Jet_QSM refnum"=w80, "error in (no error)"=w77, "state(s)"=w79) -> ("error out"=w78:errorcluster)  [unwired: 8 in]
          }
          frame "Error Handler" {
            n60 = Bundle By Name(cluster=w197, "error"=w198) -> (w196:refnum<class "Module_UI_TopLevel.lvclass">)
            n61 = Get Date/Time In Seconds() -> (seconds since 1Jan1904=w206:timestamp)
            n62 = call <userlib>:"JET_QSM - Flush Debug Queue.vi"("Jet_QSM refnum"=w202) -> ("QSM Elements"=w204:T13[], "Timestamps"=w205:timestamp[])  [unwired: 8 in, 1 out]
            n63 = Unbundle By Name(w198) -> ("code"=w199:i32)
            n64 = for {
              tunnel: w204 -> [w218] mode=indexing
              tunnel: [w216] -> w208 mode=indexing
              tunnel: w206 -> [w213]
              tunnel: w205 -> [w214] mode=indexing
              n65 = Subtract(x=w213, y=w214) -> (x-y=w212:dbl)
              n66 = To Double Precision Float(number=w212) -> (double precision float=w211:dbl)
              n67 = Unbundle By Name(w218) -> ("state"=w217:string)
              n68 = Format Into String(format string="%.03f sec ago: %s", w211, w217) -> (resulting string=w216:string)  [unwired: 2 in, 1 out]
            }
            n69 = case "Specific Error Code?" shown="Default" w199 {
              selector: w199 -> [w220]
              tunnel: [w221] -> w200
              tunnel: w198 -> [w219]
              frame Default {
                w221 = TRUE  # Exit?
                n70 = call <vilib>:"Simple Error Handler.vi"("error code (no error:0)"=w220, "error in (no error)"=w219) -> ()  [unwired: 3 in, 5 out]
              }
            }
            n71 = Array To Spreadsheet String(delimiter (Tab)="\n", array=w208, 3:"%s" ("format string")) -> (spreadsheet string=→"Recent states before Error (with tick counts) 2":string)
            n72 = call-poly <userlib>:"JET_QSM - Add State(s).vi"("act? (T)"=w200, "Jet_QSM refnum"=w202, "state(s)"="VI Exit") -> ("error out"=w203:errorcluster)  [unwired: 8 in]
          }
          frame "VI Exit" {
            n73 = flat-sequence {
              tunnel: w229 -> [w235]
              tunnel: w228 -> [w234]
              tunnel: [w234] -> w227
              tunnel: w227 -> [w237]
              tunnel: [w237] -> w224
              tunnel: w224 -> [w238]
              frame #0 {
                n74 = call <userlib>:"JET_QSM - Flush.vi"("Jet_QSM ref"=w234, "error in (no error)"=w235) -> ()  [unwired: 8 in, 2 out]
              }
              frame #1 {
                w236 = "Window: Close\nControl Update"  # Exiting Process
                n75 = call-poly <userlib>:"JET_QSM - Add State(s).vi"("Jet_QSM refnum"=w237, "state(s)"=w236) -> ()  [unwired: 9 in, 1 out]
              }
              frame #2 {
                n76 = call <userlib>:"JET_QSM - Add STOP.vi"("Jet_QSM refnum"=w238) -> ()  [unwired: 10 in, 1 out]
              }
            }
            n77 = disable-structure shown="Enabled" {
              disable-tunnel: w223 -> [w232 w233]
              disable-tunnel: [w231 w233] -> w222
              frame Enabled {
                n78 = call <userlib>:"(create) jMsg_JSMA_ApplicationShutdown.vi"() -> ("jMsg_JSMA_ApplicationShutdown"=w230:refnum<class "jMsg_JSMA_ApplicationShutdown.lvclass">)  [unwired: 10 in, 1 out]
                n79 = call <userlib>:"jModule - MessageTx.vi"("jMsg"=w230, "jModule"=w232) -> ("jModule"=w231:refnum<class "Module_UI_TopLevel.lvclass">)  [unwired: 6 in, 3 out]
              }
              frame Disabled {
              }
            }
            n80 = Bundle By Name(cluster=w222, "isExiting?"=TRUE ("VI.isExiting?")) -> (w226:refnum<class "Module_UI_TopLevel.lvclass">)
          }
          frame "VI STOP" {
            # "Pass out any error that was cached"
            # "This State is the STOP State.\nIt ALWAYS is the last state to execute."
            n81 = call-dynamic "Destroy.vi"("JETPanel in"=w240) -> ()  [unwired: 10 in, 1 out]
            n82 = Unbundle By Name(w239) -> ("error"=w241:errorcluster)
            n83 = call-dynamic "jModule - Destroy.vi"("jModule"=w239) -> ()  [unwired: 10 in, 1 out]
          }
          frame "INVALID STATE", Default {
            # "This is the state that handles a state name that is INVALID (there is no state for it in the state machine)"
            n84 = call-dynamic "jModule - Handle Invalid MessageRx.vi"("error in (no error)"=w247, "Invalid State"=w246, "jModule"=w243) -> ("error out"=w250:errorcluster, "is jMsg State?"=w248:bool, "Invalid State"=w249:string, "jModule"=w242:refnum<class "Module_UI_TopLevel.lvclass">)  [unwired: 5 in]
            n85 = case "is jMsg?" shown="False" w248 {
              tunnel: [w254 w255] -> w245
              tunnel: w250 -> [w253 w255]
              tunnel: w249 -> [w252 _]
              tunnel: w244 -> [w251 _]
              frame False {
                n86 = call <userlib>:"JET_QSM - INVALID State.vi"("Jet_QSM refnum"=w251, "error in (no error)"=w253, "state"=w252) -> ("error out"=w254:errorcluster)  [unwired: 8 in]
              }
              frame True {
              }
            }
          }
          frame "------ Menu Commands ------" {
            # "This is a section header; the state is never expected to execute"
          }
          frame "------ jMsg  ------" {
            # "This is a section header; the state is never expected to execute"
          }
          frame "jMsg_JSMA_ApplicationShutdown" {
            n87 = call-poly <userlib>:"JET_QSM - Add State(s).vi"("Jet_QSM refnum"=w264, "error in (no error)"=w260, "state(s)"="VI Exit") -> ("error out"=w263:errorcluster)  [unwired: 8 in]
          }
          frame "jMsg_GUISubPanel_Dock" {
            # "It is done this way so that Subpanel UIs can pass control to one another..."
            n88 = call <userlib>:"jMsg_Sys_GUIPanelDock - Rx Read.vi"("jModule"=w266) -> ("SubPanelControl.refnum"=w268:refnum<vi>, "GUISubPanel Module"=w267:string, "jModule"=w265:refnum<class "Module_UI_TopLevel.lvclass">)  [unwired: 5 in, 3 out]
            n89 = Unbundle By Name(w265) -> ("refnum"=w274:refnum<vi>, "refnum"=w273:refnum<vi>, "refnum"=w272:refnum<vi>)
            n90 = Build Array(w274, w273, w272) -> (w271:refnum<vi>[])
            n91 = Search 1D Array(1D array=w271, element=w268) -> (index of element=w270:i32)  [unwired: 1 in]
            n92 = case shown="1" w270 {
              tunnel: w265 -> [w278 w284 w290 w294]
              tunnel: [w277 w283 w289 w294] -> w269
              tunnel: w267 -> [w276 w282 w288 _]
              frame 1 {
                n93 = in-place {
                  in-place-border: w276 -> [w281]
                  n94 = in-place-cluster #1(w278) -> ("ActivePanel"=w280:T2)
                  n95 = Scan From String(input string=w281, default 1=w280) -> (output 1=w279:T2)  [unwired: 3 in, 3 out]
                  n96 = in-place-cluster #1("ActivePanel"=w279) -> (w277:refnum<class "Module_UI_TopLevel.lvclass">)
                }
              }
              frame 2 {
                n97 = in-place {
                  in-place-border: w282 -> [w287]
                  n98 = in-place-cluster #2(w284) -> ("ActivePanel"=w286:T3)
                  n99 = Scan From String(input string=w287, default 1=w286) -> (output 1=w285:T3)  [unwired: 3 in, 3 out]
                  n100 = in-place-cluster #2("ActivePanel"=w285) -> (w283:refnum<class "Module_UI_TopLevel.lvclass">)
                }
              }
              frame 0 {
                n101 = in-place {
                  in-place-border: w288 -> [w293]
                  n102 = in-place-cluster #3(w290) -> ("ActivePanel"=w292:T1)
                  n103 = Scan From String(input string=w293, default 1=w292) -> (output 1=w291:T1)  [unwired: 3 in, 3 out]
                  n104 = in-place-cluster #3("ActivePanel"=w291) -> (w289:refnum<class "Module_UI_TopLevel.lvclass">)
                }
              }
              frame Default {
              }
            }
          }
          frame "jMsg_Sys_UIPanel_Open" {
            n105 = call <userlib>:"jMsg_Sys_UIPanel_Open - Rx Read.vi"("error in (no error)"=w297, "jModule"=w298) -> ("error out"=w296:errorcluster, "UI Name"=w299:string, "jModule"=w295:refnum<class "Module_UI_TopLevel.lvclass">)  [unwired: 5 in, 2 out]
            n106 = Equal?(x=w299, y=w301) -> (x = y?=w300:bool)
            n107 = call-poly <userlib>:"JET_QSM - Add State(s).vi"("act? (T)"=w300, "Jet_QSM refnum"=w304, "error in (no error)"=w296, "state(s)"="Window: Open") -> ("error out"=w303:errorcluster)  [unwired: 7 in]
          }
          frame "jMsg_Sys_VersionInfo" {
            n108 = call <userlib>:"jMsg_Sys_VersionInfo - Rx Read.vi"("jModule"=w306) -> ("VersionInfo"=w307:T14, "jModule"=w305:refnum<class "Module_UI_TopLevel.lvclass">)  [unwired: 7 in, 2 out]
            n109 = call <userlib>:"jSWCfg - Add New VersionInfo.vi"("VersionInfo"=w307) -> ()  [unwired: 10 in, 1 out]
            n110 = Unbundle By Name(w307) -> ("ID"=→"String":string)
            n111 = call-poly <userlib>:"JET_QSM - Add State(s).vi"("Jet_QSM refnum"=w312, "error in (no error)"=w310, "state(s)"="SoftwareConfig: Update") -> ("error out"=w309:errorcluster)  [unwired: 8 in]
          }
          frame "jMsg_TCP_Connected" {
            n112 = Bundle By Name(cluster=w319, "TCPConnected?"=TRUE ("connected?")) -> (w318:refnum<class "Module_UI_TopLevel.lvclass">)
            n113 = call-poly <userlib>:"JET_QSM - Add State(s).vi"("Jet_QSM refnum"=w314, "error in (no error)"=w317, "state(s)"="Indicator Update") -> ("error out"=w316:errorcluster)  [unwired: 8 in]
          }
          frame "jMsg_TCP_Disconnected" {
            n114 = Bundle By Name(cluster=w326, "TCPConnected?"=FALSE ("connected?")) -> (w325:refnum<class "Module_UI_TopLevel.lvclass">)
            n115 = call-poly <userlib>:"JET_QSM - Add State(s).vi"("Jet_QSM refnum"=w321, "error in (no error)"=w324, "state(s)"="Indicator Update") -> ("error out"=w323:errorcluster)  [unwired: 8 in]
          }
          frame "------ Actions  ------" {
            # "This is a section header; the state is never expected to execute"
          }
          frame "Debug: Show" {
            n116 = call <userlib>:"(create) jMsg_Sys_UIPanel_Open.vi"("UI Name"="DebugUI" ("GUI")) -> ("jMsg_Sys_UIPanel_Open"=w330:refnum<class "jMsg_Sys_UIPanel_Open.lvclass">)  [unwired: 10 in]
            n117 = call <userlib>:"jModule - MessageTx.vi"("error in (no error)"=w334, "jMsg"=w330, "jModule"=w332) -> ("error out"=w333:errorcluster, "jModule"=w331:refnum<class "Module_UI_TopLevel.lvclass">)  [unwired: 5 in, 2 out]
          }
          frame "Menu: Button Command" {
            # "This is here so the software can command a button press"
            n118 = Unbundle By Name(w340) -> ("refnum"=w338:refnum<vi>, "ButtonPressed"=w339:string)
            n119 = property class="Menu Button (strict)"(reference=w338) -> (reference out=w336:refnum<vi>, "Value"=w337:T4)  [unwired: 1 in, 1 out]
            n120 = Bundle By Name(cluster=w337, "Button Pressed"=w339) -> (w335:T4)
            n121 = property class="Menu Button (strict)"(reference=w336, "Value"=w335) -> ()  [unwired: 1 in, 2 out]
          }
          frame "Menu: Initialize" {
            n122 = Unbundle By Name(w350) -> ("refnum"=w349:refnum<vi>)
            n123 = Build Path(base path=w351, name or relative path="MenuConfig.ini") -> (appended path=w348:path)
            n124 = invoke class="Menu Button (strict)" method="Configure Button from File.vi"(reference=w349, error in=w347, "Configuration Path"=w348) -> (reference out=w346:refnum<vi>, error out=w344:errorcluster)  [unwired: 3 in, 4 out]
            n125 = property class="Menu Button (strict)"(reference=w346) -> ("Value"=w345:T4)  [unwired: 1 in, 2 out]
            n126 = Unbundle By Name(w345) -> ("Button Pressed"=w343:string, "Level"=w342:string)
            n127 = Bundle By Name(cluster=w350, "ButtonPressed"=w343, "Level"=w342) -> (w353:refnum<class "Module_UI_TopLevel.lvclass">)
          }
          frame "SubPanel: Center Dock" {
            n128 = Unbundle By Name(w354) -> ("ActivePanel"=w358:T1, "refnum"=w359:refnum<vi>)
            "Center" <- w358
            n129 = Format Into String(w358) -> (resulting string=w357:string)  [unwired: 3 in, 1 out]
            n130 = call <userlib>:"(create) jMsg_Sys_GUIPanelDock.vi"("Owner jModule"=w354, "SubPanelControl.refnum"=w359, "GUISubPanel Module"=w357) -> ("jMsg_GUISubPanel_Dock"=w356:refnum<class "jMsg_GUISubPanel_Dock.lvclass">)  [unwired: 7 in, 1 out]
            n131 = call <userlib>:"jModule - MessageTx.vi"("jMsg"=w356, "jModule"=w354) -> ("jModule"=w355:refnum<class "Module_UI_TopLevel.lvclass">)  [unwired: 6 in, 3 out]
          }
          frame "SubPanel: Bottom Dock" {
            n132 = Unbundle By Name(w361) -> ("ActivePanel"=w365:T2, "refnum"=w366:refnum<vi>)
            "Bottom" <- w365
            n133 = Format Into String(w365) -> (resulting string=w364:string)  [unwired: 3 in, 1 out]
            n134 = call <userlib>:"(create) jMsg_Sys_GUIPanelDock.vi"("Owner jModule"=w361, "SubPanelControl.refnum"=w366, "GUISubPanel Module"=w364) -> ("jMsg_GUISubPanel_Dock"=w363:refnum<class "jMsg_GUISubPanel_Dock.lvclass">)  [unwired: 7 in, 1 out]
            n135 = call <userlib>:"jModule - MessageTx.vi"("jMsg"=w363, "jModule"=w361) -> ("jModule"=w362:refnum<class "Module_UI_TopLevel.lvclass">)  [unwired: 6 in, 3 out]
          }
          frame "SubPanel: Right Dock" {
            (unwired) Module_UI_TopLevel_SPRight_STYP."Module_SP_RightBlank#7"  # my.UI.SP_right.ActivePanel
            n136 = Unbundle By Name(w368) -> ("ActivePanel"=w372:T3, "refnum"=w370:refnum<vi>)
            "Right" <- w372
            n137 = Format Into String(w372) -> (resulting string=w371:string)  [unwired: 3 in, 1 out]
            n138 = call <userlib>:"(create) jMsg_Sys_GUIPanelDock.vi"("Owner jModule"=w368, "SubPanelControl.refnum"=w370, "GUISubPanel Module"=w371) -> ("jMsg_GUISubPanel_Dock"=w369:refnum<class "jMsg_GUISubPanel_Dock.lvclass">)  [unwired: 7 in, 1 out]
            n139 = call <userlib>:"jModule - MessageTx.vi"("jMsg"=w369, "jModule"=w368) -> ("jModule"=w373:refnum<class "Module_UI_TopLevel.lvclass">)  [unwired: 6 in, 3 out]
          }
          frame "------ Window and Panel Control ------" {
            # "This is a section header; the state is never expected to execute"
          }
          frame "SoftwareConfig: Update" {
            n140 = call <userlib>:"jSWCfg - Get VersionInfo.vi"("Component List"=string[] ["Host", "FPGA"]) -> ("VersionInfo[]"=w377:T15[])  [unwired: 10 in]
            n141 = for {
              tunnel: w377 -> [w383] mode=indexing
              n142 = Unbundle By Name(w383) -> ("target ID"=w382:string, "version"=w381:string)
              n143 = case shown="\"Host\"" w382 {
                tunnel: w381 -> [_ w386 w389]
                frame Default {
                }
                frame "Host" {
                  n144 = Format Into String(format string="v%s", w386) -> (resulting string=→"Host":string)  [unwired: 2 in, 1 out]
                }
                frame "FPGA" {
                  n145 = Format Into String(format string="v%s", w389) -> (resulting string=→"FPGA":string)  [unwired: 2 in, 1 out]
                }
              }
            }
          }
          frame "Control Update" {
            n146 = call-poly <userlib>:"JET_QSM - Add State(s).vi"("Jet_QSM refnum"=w394, "error in (no error)"=w393, "state(s)"="Indicator Update") -> ("error out"=w392:errorcluster)  [unwired: 8 in]
            n147 = disable-structure shown="Disabled" {
              frame Disabled {
                n148 = call <userlib>:"VI Control - Disable Control.vi"() -> ("Disabled Attribute"=w395:T16)  [unwired: 8 in, 1 out]
                n149 = property on="exit?" class="Bool"("DisabledEnum"=w395) -> ()  [unwired: 2 in, 2 out]
              }
              frame Enabled {
              }
            }
          }
          frame "Indicator Update" {
            n150 = Unbundle By Name(w396) -> ("TCPConnected?"=→"JETLogo":bool)
            n151 = disable-structure shown="Disabled" {
              frame Disabled {
                w399 = 0  # Dropped Connections
                w400 = 0  # Connections Made
                w401 = 0  # Connection Attempts
                n152 = Format Into String(format string="%d-%d-%d", w401, w400, w399) -> (resulting string=→"TCPStats":string)  [unwired: 2 in, 1 out]
              }
              frame Enabled {
              }
            }
          }
          frame "Window: Open" {
            n153 = disable-structure shown="Enabled" {
              disable-tunnel: w413 -> [w421 w422]
              disable-tunnel: [w420 w422] -> w405
              frame Disabled {
                n154 = call <userlib>:"Position.vi"("Monitor (1)"=u16 2, "JETPanel in"=w421) -> ("JETPanel out"=w420:refnum<class "JETPanel.lvclass">)  [unwired: 8 in, 1 out]
              }
              frame Enabled {
              }
            }
            n155 = call <userlib>:"jSWCfg - Get Properties.vi"() -> ("properties"=w412:T17)  [unwired: 10 in, 1 out]
            n156 = Unbundle By Name(w412) -> ("SoftwareInfo.array"=w411:T15[])
            n157 = Index Array(array=w411) -> (element=w408:T15)  [unwired: 1 in]
            n158 = call-poly <userlib>:"JET_QSM - Add State(s).vi"("Jet_QSM refnum"=w417, "error in (no error)"=w416, "state(s)"="Control Update") -> ("error out"=w415:errorcluster)  [unwired: 8 in]
            n159 = Unbundle By Name(w408) -> ("version"=w407:string)
            n160 = Format Into String(format string=" v%s", initial string=w409, w407) -> (resulting string=w406:string)  [unwired: 1 in, 1 out]
            n161 = call <userlib>:"Set Window Title.vi"("Window Title"=w406, "JETPanel in"=w405) -> ("JETPanel out"=w404:refnum<class "JETPanel.lvclass">)  [unwired: 8 in, 1 out]
            n162 = call-dynamic "PanelOpen.vi"("JETPanel in"=w404) -> ()  [unwired: 9 in, 2 out]
          }
          frame "Window: Close" {
            n163 = call-dynamic "PanelClose.vi"("JETPanel"=w423) -> ()  [unwired: 9 in, 2 out]
          }
        }
      }
      n164 = while {
        tunnel: w16 -> [w32]
        stop <- w33 stop-if-true
        n165 = call <userlib>:"jFlag_MasterShutdown - Get.vi"("error in (no error)"=w32) -> ("Shutdown?"=w33:bool)  [unwired: 9 in, 1 out]
        n166 = Get Date/Time In Seconds() -> (seconds since 1Jan1904=w35:timestamp)
        n167 = To Double Precision Float(number=w35) -> (double precision float=→"currentDateTime":dbl)
        n168 = Wait Until Next ms Multiple(millisecond multiple=u32 1000) -> ()  [unwired: 1 out]
      }
    }
    frame Error {
    }
  }
  "error out" <- w6
